vi "ASCII to Hex.vi"(1 "ASCII":string) -> (0 "Hex":string)   [LabVIEW 2014]
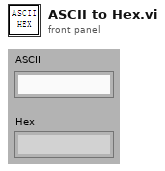
[diagram p1: front panel]
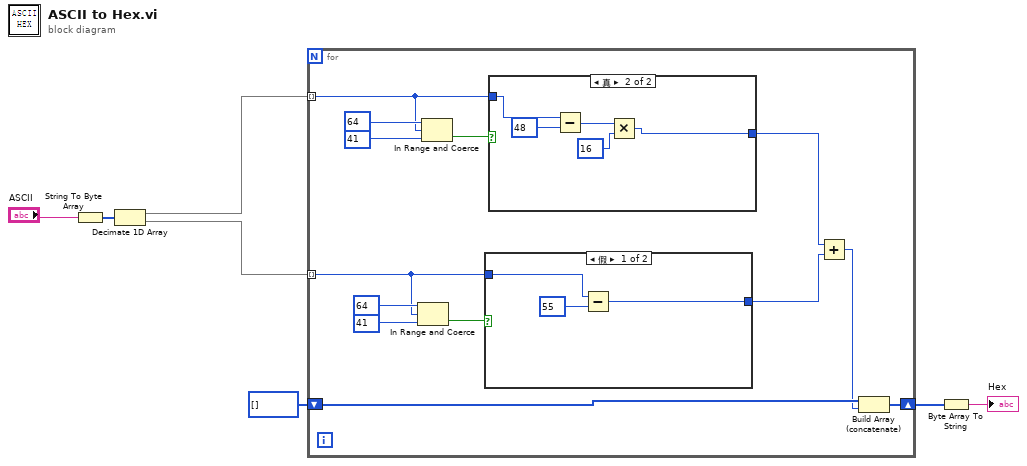
[diagram p0: block diagram]
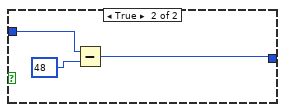
[diagram p2: hidden frame]
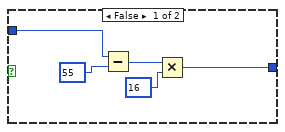
[diagram p3: hidden frame]
diagram:
  n1 = String To Byte Array(string="ASCII") -> (unsigned byte array=w3:u8[])
  n2 = Decimate 1D Array(w3) -> (w2:u8[], w1:u8[])
  n3 = for {
    shift-right: [w10] -> w6
    shift-left: u8[] [] -> [w12]
    tunnel: w2 -> [w9] mode=indexing
    tunnel: w1 -> [w8] mode=indexing
    n4 = In Range and Coerce(upper limit=u8 64 ("上限"), x=w8, lower limit=u8 41 ("下限")) -> (In Range?=w15:bool)  [unwired: 1 out]
    n5 = In Range and Coerce(upper limit=u8 64 ("上限"), x=w9, lower limit=u8 41 ("下限")) -> (In Range?=w18:bool)  [unwired: 1 out]
    n6 = case shown="假" w15 {
      tunnel: w8 -> [w21 w25]
      tunnel: [w22 w24] -> w13
      frame False {
        n7 = Subtract(x=w21, y=u8 55 ("上限")) -> (x-y=w22:u8)
      }
      frame True {
        n8 = Subtract(x=w25, y=u8 48 ("上限")) -> (x-y=w24:u8)
      }
    }
    n9 = case shown="真" w18 {
      tunnel: w9 -> [w28 w32]
      tunnel: [w27 w33] -> w14
      frame False {
        n10 = Subtract(x=w28, y=u8 55 ("上限")) -> (x-y=w30:u8)
        n11 = Multiply(x=w30, y=u8 16 ("上限")) -> (x*y=w27:u8)
      }
      frame True {
        n12 = Subtract(x=w32, y=u8 48 ("上限")) -> (x-y=w35:u8)
        n13 = Multiply(x=w35, y=u8 16 ("上限")) -> (x*y=w33:u8)
      }
    }
    n14 = Add(x=w14, y=w13) -> (x+y=w11:u8)
    n15 = Build Array (concatenate)(w12, w11) -> (w10:u8[])
  }
  n16 = Byte Array To String(unsigned byte array=w6) -> (string=→"Hex":string)
